vi "BindCluster.vi"(8 "error in (no error)":errorcluster, 9 "Controls[]":refnum<vi>[](array[refnum]), 10 "Cols":T1[](array[typedef]), 11 "SQL Statement in":refnum<class "SQL Statement.lvclass">) -> (0 "error out":errorcluster, 2 "Array":string[](array[string]), 3 "SQL Statement out":refnum<class "SQL Statement.lvclass">, 5 "Time":u32)   [LabVIEW 2017, in "Beltwatch SQLite.lvlib"]
uses:
  Beltwatch/BeltWatch 4-2-2-5/Database/Beltwatch SQLite.lvlib
  <vilib>/drjdpowell/SQLite Library/SQL Statement/SQL Statement.lvclass
  Common64/Database/SQ Lite/SQ Lite Cluster Action.ctl
  <vilib>/drjdpowell/SQLite Library/SQL Statement/SQL Statement.lvclass/SQL Statement.ctl
  <vilib>/drjdpowell/SQLite Library/SQL Statement/Bind Integer.vi
  <vilib>/drjdpowell/SQLite Library/SQL Statement/Bind Blob.vi
  <vilib>/drjdpowell/SQLite Library/SQL Statement/Bind Null.vi
  <vilib>/drjdpowell/SQLite Library/SQL Statement/Bind Real.vi
  <vilib>/drjdpowell/SQLite Library/SQL Statement/Bind Text.vi
  <vilib>/drjdpowell/SQLite Library/SQL Statement/Error Message.vi
panel:
  out "?":string
  out "Waveform Chart":u32(graph)
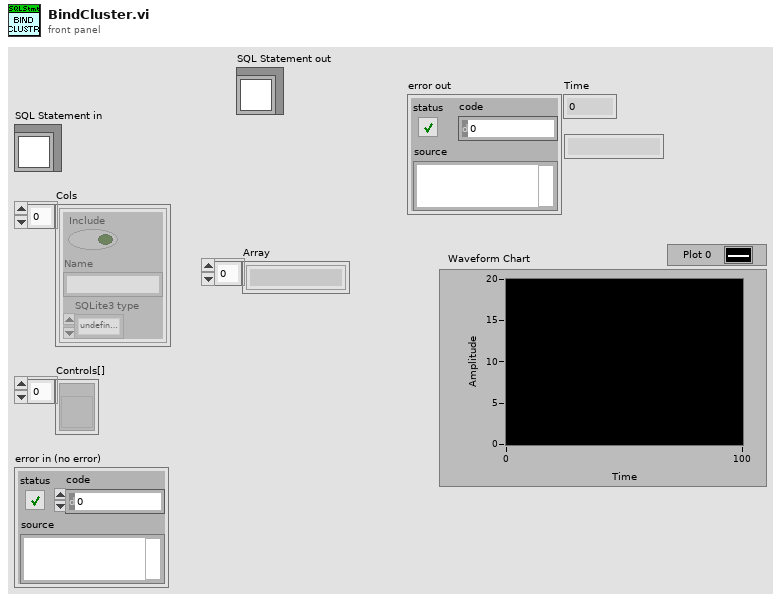
[diagram p1: front panel]
types:
  T1 = typedef "Beltwatch SQLite.lvlib/SQ Lite Cluster Action.ctl" = cluster{"Include":bool, "Name":string, "SQLite3 type":enum32{"undefined type (0)", "SQLITE_INTEGER", "SQLITE_FLOAT", "SQLITE3_TEXT", "SQLITE_BLOB", "SQLITE_NULL", "undefined type"}}
  T2 = enum32{"undefined type (0)", "SQLITE_INTEGER", "SQLITE_FLOAT", "SQLITE3_TEXT", "SQLITE_BLOB", "SQLITE_NULL", "undefined type"}
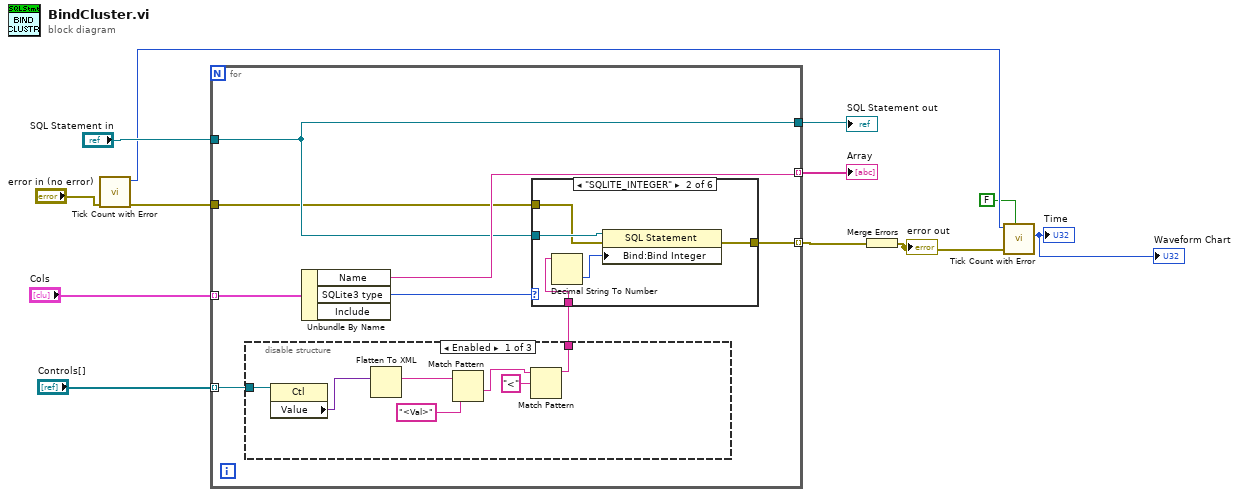
[diagram p0: block diagram]
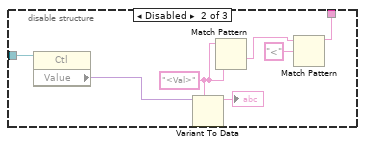
[diagram p2: hidden frame]
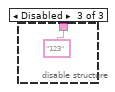
[diagram p3: hidden frame]
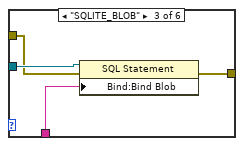
[diagram p5: hidden frame]
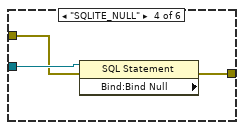
[diagram p6: hidden frame]
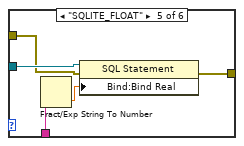
[diagram p7: hidden frame]
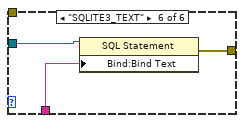
[diagram p8: hidden frame]
diagram:
  n1 = call "Tick Count with Error.vi"("error in (no error)"="error in (no error)") -> ("error out"=w5:errorcluster, "millisecond timer value"=w3:u32)  [unwired: 8 in, 1 out]
  n2 = for {
    tunnel: "Cols" -> [w20] mode=indexing
    tunnel: "Controls[]" -> [w19] mode=indexing
    tunnel: [w17] -> w9 mode=indexing
    tunnel: w5 -> [w14]
    tunnel: "SQL Statement in" -> [w15]
    tunnel: [w15] -> w12
    tunnel: [w13] -> w7 mode=indexing
    n3 = disable-structure shown="Enabled" {
      disable-tunnel: w19 -> [w27 w31 _]
      disable-tunnel: [w21 w32 "123" ("regular expression")] -> w16
      frame Enabled {
        n4 = property class="Ctl"(reference=w27) -> ("Value"=w26:variant)  [unwired: 1 in, 2 out]
        n5 = Flatten To XML(anything=w26) -> (xml string=w25:string)
        n6 = Match Pattern(string=w25, regular expression="<Val>") -> (after substring=w23:string)  [unwired: 1 in, 3 out]
        n7 = Match Pattern(string=w23, regular expression="<") -> (before substring=w21:string)  [unwired: 1 in, 3 out]
      }
      frame Disabled {
        w28 = "<Val>" ("regular expression")
        n8 = property class="Ctl"(reference=w31) -> ("Value"=w30:variant)  [unwired: 1 in, 2 out]
        n9 = Variant To Data(type=w28, Variant=w30) -> (data=→"?":string)  [unwired: 1 in, 1 out]
        n10 = Match Pattern(string=w28, regular expression=w28) -> (after substring=w34:string)  [unwired: 1 in, 3 out]
        n11 = Match Pattern(string=w34, regular expression="<") -> (before substring=w32:string)  [unwired: 1 in, 3 out]
      }
      frame Disabled {
      }
    }
    n12 = Unbundle By Name(w20) -> ("Name"=w17:string, "SQLite3 type"=w18:T2)  [unwired: 1 out]
    n13 = case shown="\"SQLITE_INTEGER\"" w18 {
      tunnel: w15 -> [_ w41 w45 w48 w53 w56]
      tunnel: w16 -> [_ w40 w44 _ w52 w55]
      tunnel: w14 -> [w36 w37 w42 w46 w50 _]
      tunnel: [w36 w38 w43 w47 w49 w54] -> w13
      frame "undefined type (0)", Default {
      }
      frame "SQLITE_INTEGER" {
        n14 = Decimal String To Number(string=w40) -> (number=w39:i32)  [unwired: 2 in, 1 out]
        n15 = property class="SQL Statement"(reference=w41, error in=w37, "Bind:Bind Integer"=w39) -> (error out=w38:errorcluster)  [unwired: 1 out]
      }
      frame "SQLITE_BLOB" {
        n16 = property class="SQL Statement"(reference=w45, error in=w42, "Bind:Bind Blob"=w44) -> (error out=w43:errorcluster)  [unwired: 1 out]
      }
      frame "SQLITE_NULL" {
        n17 = property class="SQL Statement" props=["Bind:Bind Null"](reference=w48, error in=w46) -> (error out=w47:errorcluster)  [unwired: 2 out]
      }
      frame "SQLITE_FLOAT" {
        n18 = Fract/Exp String To Number(string=w52) -> (number=w51:dbl)  [unwired: 3 in, 1 out]
        n19 = property class="SQL Statement"(reference=w53, error in=w50, "Bind:Bind Real"=w51) -> (error out=w49:errorcluster)  [unwired: 1 out]
      }
      frame "SQLITE3_TEXT" {
        n20 = property class="SQL Statement"(reference=w56, "Bind:Bind Text"=w55) -> (error out=w54:errorcluster)  [unwired: 1 in, 1 out]
      }
    }
  }
  "SQL Statement out" <- w12
  "Array" <- w9
  n21 = Merge Errors(w7) -> (w4:errorcluster)
  "error out" <- w4
  n22 = call "Tick Count with Error.vi"("UsePrevious"=FALSE, "error in (no error)"=w4, "millisecond val in"=w3) -> ("Time"=→"Time" →"Waveform Chart":u32)  [unwired: 6 in, 2 out]
